vi "GT Set Laser Dis Table1D.vi"(0 "cardNum":i16, 1 "minPower":dbl, 2 "pLimitPower":dbl, 5 "count":i16, 7 "pRatio":dbl, 9 "pPos":i32, 11 "error in (no error)":errorcluster caption="错误输入（无错误）", 12 "maxPower":dbl, 13 "channel":i16) -> (4 "pLimitPower out":dbl, 6 "function return":i16, 8 "pRatio out":dbl, 10 "pPos out":i32, 15 "error out":errorcluster caption="错误输出")   [LabVIEW 2020, in "gts.lvlib"]
doc: "GT_API GT_SetLaserDisTable1D(short cardNum,short count,double *pRatio,long *pPos,double minPower,double maxPower,double *pLimitPower,short channel=0);"
uses:
  gts.lvlib
  dll/32bit/multi_card/gts.dll
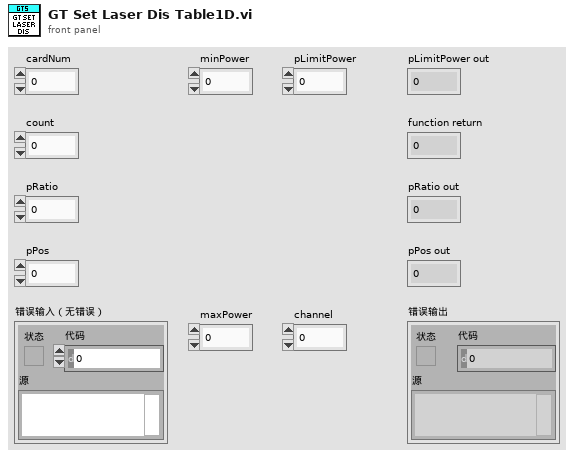
[diagram p1: front panel]
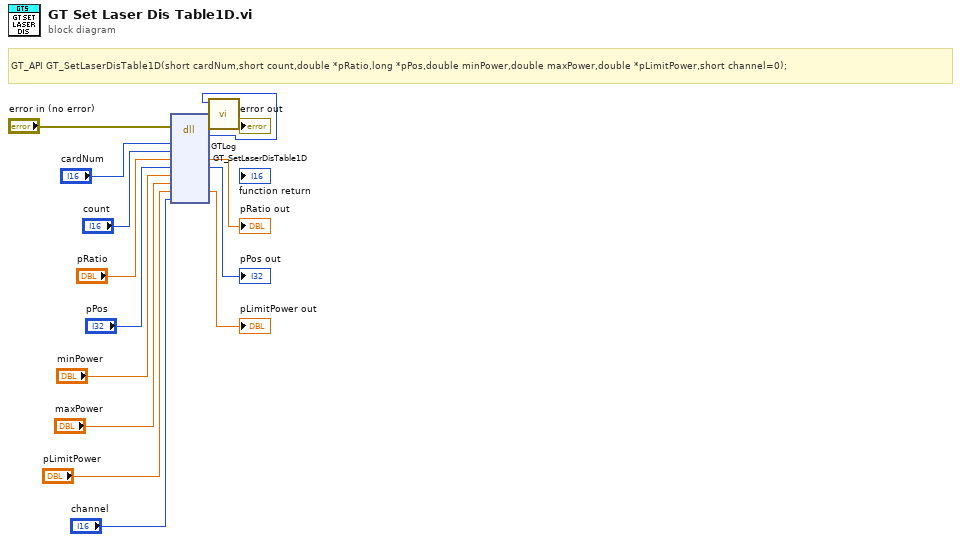
[diagram p0: block diagram]
diagram:
  # "GT_API GT_SetLaserDisTable1D(short cardNum,short count,double *pRatio,long *pPos,double minPower,double maxPower,double *pLimitPower,short channel=0);"
  n1 = dll-call lib="C:/1228/dll/32bit/multi_card/gts.dll" fn="GT_SetLaserDisTable1D"(error in="error in (no error)", "cardNum"="cardNum", "count"="count", "pRatio"="pRatio", "pPos"="pPos", "minPower"="minPower", "maxPower"="maxPower", "pLimitPower"="pLimitPower", "channel"="channel") -> (error out=w3:errorcluster, w1:i16, "pRatio"=→"pRatio out":dbl, "pPos"=→"pPos out":i32, "pLimitPower"=→"pLimitPower out":dbl)  [unwired: 7 in, 1 out]
  n2 = call "GTLog.vi"("error in (no error)"=w3, "Numeric"=w1) -> ("error out"=→"error out":errorcluster)  [unwired: 9 in]
